vi "MIMIC Commands Rev 4.vi"(6 "MIMIC HOST COMMAND":T2(ring)=enum."Read Serial Number", 8 "Input String Data Array":string[](array[string])=["1"], 9 "HWHSflag":bool, 10 "wait (ms)":u32=500, 11 "VISA resource name":refnum<visa-resource-name>="COM5") -> (0 "error out":errorcluster={"status"=FALSE, "code"=1073676294, "source"="VISA Read in MIMIC RecvCommand.vi->MIMIC Commands Rev 2.vi"}, 1 "Receive_buffer":u8[](array[numeric]) format="%x", 2 "Receive_Unpacked_Data":T1)   [LabVIEW 2014]
panel:
  out "local":i32
  out "GUID":string
  out "Array":u8[](array[numeric]) format="%x"
  out "TimeToDecode":u16
  out "VISA resource name OUT":refnum<visa-resource-name>="COM5"
  out "hex integer string":string[](array[string])=["4", "D0", "0", "0", "FF", "2C"]
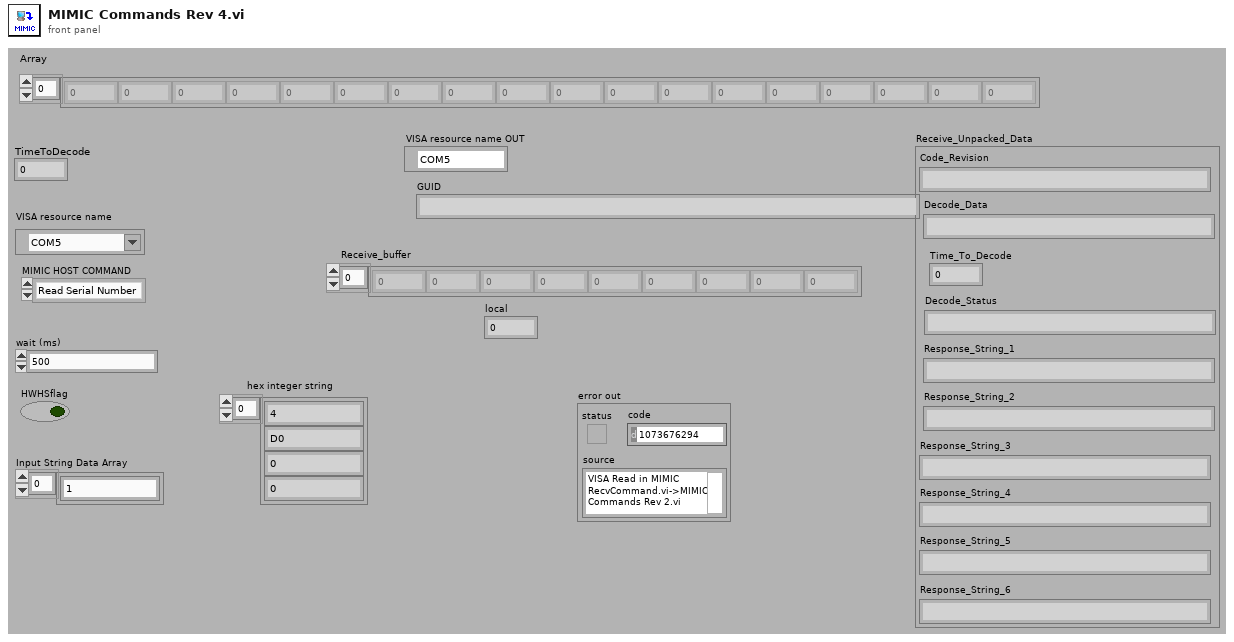
[diagram p1: front panel]
types:
  T1 = cluster{"Code_Revision":string, "Decode_Data":string, "Decode_Status":string, "Response_String_1":string, "Response_String_2":string, "Response_String_3":string, "Response_String_4":string, "Response_String_5":string, "Response_String_6":string, "Time_To_Decode":u16}
  T2 = enum16{"Enter FAT", "Beeper Control", "LED Off", "LED On", "Image Mode", "Start Session", "Stop Session", "Change Buadrate", "Auto Exposure", "Set Manual Exposure", "Read BT Address", "Store BT Address", "Pairing Command", "Query Paired Address", "Pairing Status", "Un-Pairing", "Set Illumination", "Trigger", "Set Defaults", "Imager Time To Decode Test", "Battery Off", "Battery Charge Control", "Read Battery Voltage", "Read Battery Temperature", "Software Version", "StoreFeatureSet", "ReadFeatureSet", "Store Model Number", "Read Model Number", "Store Manufacturing Date", "Read Manufacturing Date", "Store Service Date", "Read Service Date", "Store Serial Number", "Read Serial Number", "Exit FAT", "Read GUID", "Cable Auto ID", "Store RSM 627", "Read RSM 627", "Hall Effect switch", "Store GUID ", "ParamSend", "General", "General-Response", "RSM Init", "RSM EnterFAT", "RSM - SE4500 - Peek PRISM Register GENERIC command", "RSM - SE4500 - Poke PRISM Register GENERIC command", "RSM - SE4500 - GENERIC command", "RSM - SE4500 - GetPDM Calibration", "RSM - SE4500 - SetPDM Calibration", "Get Object Sensor Value", "Store Object Sensor Calibration Value", "Read Object Sensor Calibration Value", "RSM - SE4500 - GetPDM-Z Calibration", "RSM - SE4500 - SetPDM-Z Calibration"}
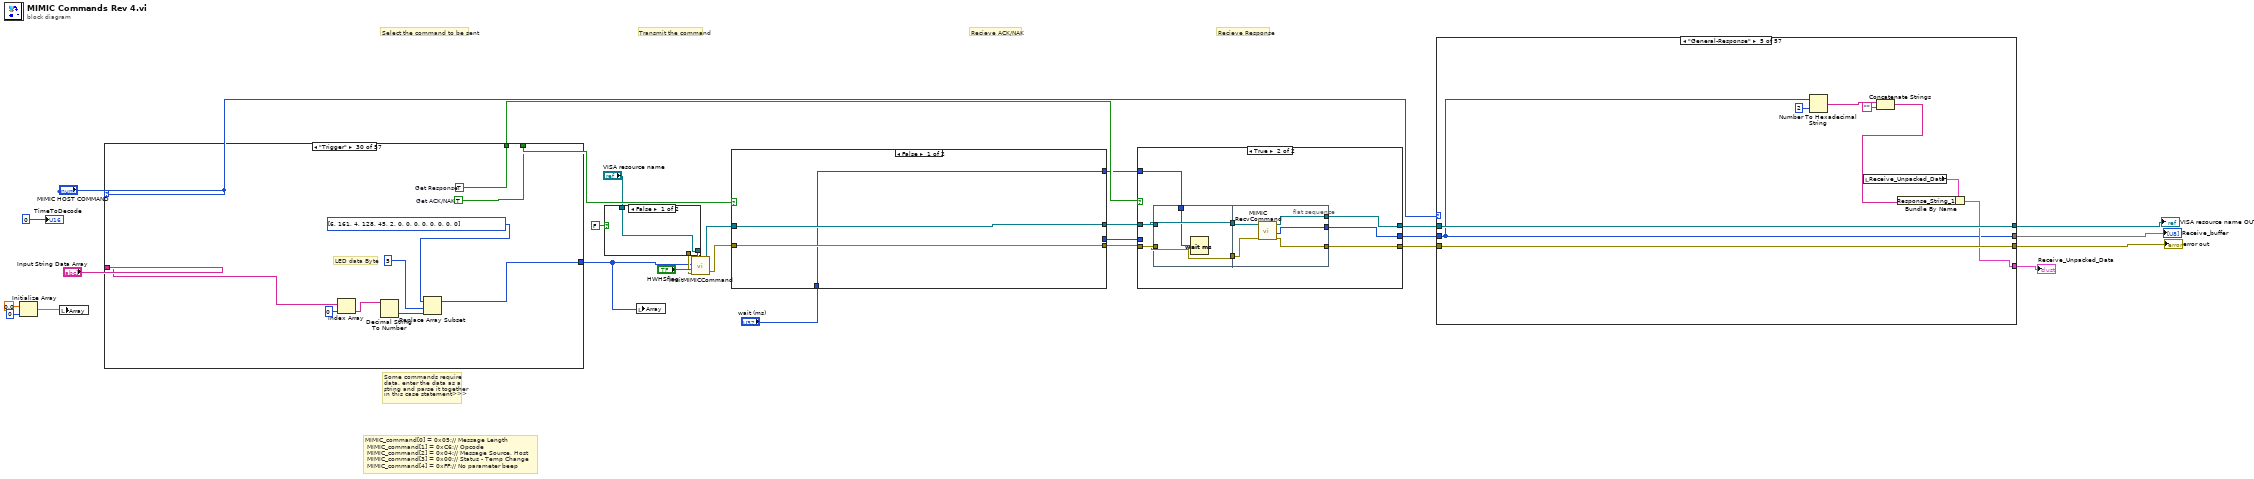
[diagram p0: block diagram]
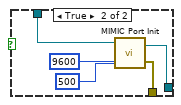
[diagram p2: hidden frame]
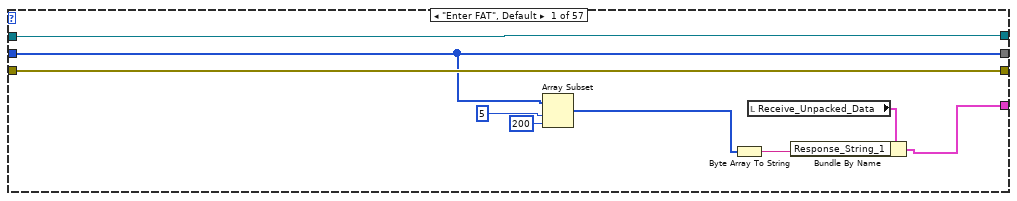
[diagram p3: hidden frame]
diagram:
  # "MIMIC_command[0] = 0x05;// Message Length \n\tMIMIC_command[1] = 0xC6;// Opcode  \n\tMIMIC_command[2] = 0x04;// Message Source, Host \n\tMIMIC_command[3] = 0x00;// Status - Temp Change            \n\tMIMIC_command[4] = 0xFF;// No parameter beep"
  # "Transmit the command"
  # "Recieve Response"
  # "Recieve ACK/NAK"
  # "Select the command to be sent"
  # "Some commands require\ndata, enter the data as a\nstring and parse it together\nin this case statement>>>"
  n1 = Initialize Array(0.0 ("element"), 0 ("dimension size")) -> (w5:dbl[])
  n2 = local write "Array"(w5) -> ()
  n3 = case shown="\"Trigger\"" "MIMIC HOST COMMAND" {
    tunnel: "Input String Data Array" -> [w37 w39 w62 _ _ _ _ _ w86 w113 w139 w179 w219 w256 _ _ _ w274 w290 w300 w313 w331 w347 _ _ _ _ _ w371 w379 _ _ w397 _ _ _ _ w422 _ w434 _ w444 _ _ _ w470 _ w482 _ _ _ _ _ _ _ _ _]
    tunnel: [w31 w45 w66 u8[] [5, 161, 4, 128, 16, 0, 0, 0, 0, 0, 0, 0, 0, 0] u8[] [14, 128, 4, 0, 0, 10, 112, 0, 1, 20, 112, 12, 0, 132] u8[] [14, 128, 4, 0, 0, 10, 112, 0, 1, 20, 112, 31, 0, 113] u8[] [12, 128, 4, 0, 0, 6, 32, 0, 0, 240, 0, 0, 0, 0] u8[] [13, 128, 4, 0, 0, 9, 112, 0, 1, 2, 120, 1, 135, 0] w85 w119 w140 w176 w217 w257 u8[] [4, 228, 4, 0, 0, 0, 0, 0, 0, 0, 0, 0, 0, 0] u8[] [4, 228, 4, 0, 0, 0, 0, 0, 0, 0, 0, 0, 0, 0] u8[] [7, 215, 4, 0, 4, 11, 0, 255, 15, 0, 0, 0, 0, 0] w275 w284 w298 w317 w334 w346 u8[] [16, 161, 4, 128, 16, 0, 0, 0, 0, 0, 0, 0, 0, 0] u8[] [5, 161, 4, 128, 16, 0, 0, 0, 0, 0, 0, 0, 0, 0] u8[] [4, 200, 4, 128, 0, 0, 0, 0, 0, 0, 0, 0, 0, 0] u8[] [5, 161, 4, 128, 25, 0, 0, 0, 0, 0, 0, 0, 0, 0] u8[] [7, 161, 4, 128, 66, 2, 29, 0, 0, 0, 0, 0, 0, 0] w370 w381 u8[] [7, 161, 4, 128, 48, 19, 136, 0, 0, 0, 0, 0, 0, 0] u8[] [5, 161, 4, 128, 60, 0, 0, 0, 0, 0, 0, 0, 0, 0] w396 u8[] [7, 161, 4, 128, 66, 117, 48, 0, 0, 0, 0, 0, 0, 0] u8[] [7, 161, 4, 128, 66, 117, 49, 0, 0, 0, 0, 0, 0, 0] u8[] [7, 161, 4, 128, 66, 78, 41, 0, 0, 0, 0, 0, 0, 0] u8[] [6, 161, 4, 128, 96, 8] w415 u8[] [7, 161, 4, 128, 66, 3, 36] w436 u8[] [7, 161, 4, 128, 66, 2, 194, 0, 0, 0, 0, 0, 0, 0] w449 u8[] [7, 161, 4, 128, 66, 2, 21, 0, 0, 0, 0, 0, 0, 0] w463 u8[] [7, 161, 4, 128, 66, 2, 23, 0, 0, 0, 0, 0, 0, 0] w475 u8[] [7, 161, 4, 128, 66, 2, 24, 0, 0, 0, 0, 0, 0, 0] w487 u8[] [7, 161, 4, 128, 66, 2, 22, 0, 0, 0, 0, 0, 0, 0] u8[] [5, 161, 4, 128, 54, 254, 160, 0, 0, 0, 0, 0, 0, 0] u8[] [5, 161, 4, 128, 84, 0, 0, 0, 0, 0, 0, 0, 0, 0] u8[] [5, 161, 4, 128, 47] w502 u8[] [5, 161, 4, 128, 110] u8[] [10, 161, 4, 128, 69, 2, 115, 66, 7, 2] u8[] [6, 161, 4, 128, 45, 1, 0, 0, 0, 0, 0, 0, 0, 0] u8[] [7, 161, 4, 128, 66, 2, 115]] -> w6
    tunnel: [w30 w57 w64 w71 w75 w78 w81 w84 w108 w135 w172 w192 w232 w258 w266 w269 w271 w276 w291 w301 w318 w335 w353 w356 w358 w361 w365 w369 w373 w386 w390 w393 w394 w405 w408 w410 w413 w428 w431 w439 w442 w448 w453 w462 w467 w474 w478 w485 w490 w494 w498 w499 w507 w509 w512 w515 w519] -> w25
    tunnel: [w29 w56 w65 w70 w74 w77 w80 w83 w107 w134 w171 w191 w231 w259 w267 w270 w272 w277 w292 w302 w319 w336 w354 w357 w359 w362 w364 w368 w372 w387 w389 w392 w395 w404 w407 w409 w412 w427 w430 w438 w441 w447 w454 w461 w466 w473 w479 w486 w491 w493 w497 w500 w508 w510 w513 w516 w518] -> w27
    frame "LED On" {
      w30 = FALSE  # Get Response
      w29 = TRUE  # Get ACK/NAK
      # "LED data Byte"
      n4 = Index Array(array=w37, index=0) -> (element=w36:string)
      n5 = Decimal String To Number(string=w36) -> (number=w35:i32)  [unwired: 2 in, 1 out]
      n6 = Replace Array Subset(array=u8[] [5, 231, 4, 128, 1, 0, 0, 0, 0, 0, 0, 0, 0, 0], new element=w35, index=4) -> (w31:u8[])
    }
    frame "ParamSend" {
      w57 = FALSE  # Get Response
      w56 = TRUE  # Get ACK/NAK
      n7 = Array Size(array=w39) -> (size(s)=w38:i32)
      n8 = Index Array(array=w39, index=0) -> (element=w61:string)
      n9 = Add(x=w38, y=5) -> (x+y=w43:i32)
      n10 = Hexadecimal String To Number(string=w61) -> (number=w42:u32)  [unwired: 2 in, 1 out]
      n11 = Replace Array Subset(array=u8[] [5, 198, 4, 128, 255, 0, 0, 0, 0, 0, 0, 0, 0, 0], new element=w43, index=0) -> (w54:u8[])
      n12 = Replace Array Subset(array=w54, new element=w42, index=5) -> (w50:u8[])
      n13 = Index Array(array=w39, index=2) -> (element=w49:string)
      n14 = Index Array(array=w39, index=1) -> (element=w53:string)
      n15 = Hexadecimal String To Number(string=w49) -> (number=w40:u32)  [unwired: 2 in, 1 out]
      n16 = Hexadecimal String To Number(string=w53) -> (number=w41:u32)  [unwired: 2 in, 1 out]
      n17 = Replace Array Subset(array=w50, new element=w41, index=6) -> (w46:u8[])
      n18 = Replace Array Subset(array=w46, new element=w40, index=7) -> (w45:u8[])
    }
    frame "Beeper Control" {
      w64 = FALSE  # Get Response
      w65 = TRUE  # Get ACK/NAK
      # "Beeper data Byte"
      n19 = Decimal String To Number(string=w62, offset=0) -> (number=w69:i32[])  [unwired: 1 in, 1 out]
      n20 = Replace Array Subset(array=u8[] [5, 230, 4, 128, 0, 0, 0, 0, 0, 0, 0, 0, 0, 0], new element=w69, index=4) -> (w66:u8[])
    }
    frame "Enter FAT" {
      w71 = TRUE  # Get Response
      w70 = TRUE  # Get ACK/NAK
      # "Enter FAT command:\n0x05:0xA1:0x40:0x80:0x10"
    }
    frame "RSM - SE4500 - GetPDM Calibration" {
      w75 = TRUE  # Get Response
      w74 = FALSE  # Get ACK/NAK
      # "RSM GetDPMCalibration Command"
    }
    frame "RSM - SE4500 - GetPDM-Z Calibration" {
      w78 = TRUE  # Get Response
      w77 = FALSE  # Get ACK/NAK
      # "RSM GetDPMCalibration Command"
    }
    frame "RSM Init" {
      w81 = TRUE  # Get Response
      w80 = FALSE  # Get ACK/NAK
      # "Init RSM command:\n0x0C:0x80:0x04:0x00:0x00:0x06:0x20:0x00:0x00:0xF0"
    }
    frame "RSM EnterFAT" {
      w84 = TRUE  # Get Response
      w83 = FALSE  # Get ACK/NAK
      # "RSM / SE4500 - Enter FAT command:\n0x0D:0x80:0x04:0x00:0x00:0x09:0x70:0x00:0x01:0x02:0x78:0x01:0x87:"
    }
    frame "RSM - SE4500 - Peek PRISM Register GENERIC command" {
      w108 = TRUE  # Get Response
      w107 = FALSE  # Get ACK/NAK
      # "Register Word - HEX String"
      # "RSM / SE4500 - Peek PRISM Register GENERIC command:\n0x0E:0x80:0x04:0x00:0x00:0x0B:0x70:0x00:0x01:0x02:0xC3:0xXX:0xXX:0xXX:0xCS"
      n21 = Index Array(array=w86, index=0) -> (element=w90:string)
      n22 = Hexadecimal String To Number(string=w90, default (0uL)=i16 0 ("default (0 I32)")) -> (number=w88:i16)  [unwired: 1 in, 1 out]
      n23 = Split Number(x=w88) -> (hi(x)=w94:u8, lo(x)=w92:u8)
      n24 = Replace Array Subset(array=u8[] [15, 128, 4, 0, 0, 11, 112, 0, 1, 3, 195, 0, 0, 0, 0], new element=w94, index=11) -> (w91:u8[])
      n25 = Replace Array Subset(array=w91, new element=w92, index=12) -> (w87:u8[])
      n26 = Array Subset(array=w87, index=10, length=3) -> (w97:u8[])
      n27 = for {
        N: 3 -> [_]
        tunnel: w97 -> [w111] mode=indexing
        shift-right: [w109] -> w103
        shift-left: u16 0 -> [w110]
        n28 = Add(x=w110, y=w111) -> (x+y=w109:u16)
      }
      n29 = Not(x=w103) -> (.not. x?=w102:u16)
      n30 = Increment(x=w102) -> (x+1=w101:u16)
      n31 = Replace Array Subset(array=w87, new element=w101, index=13) -> (w85:u8[])
    }
    frame "RSM - SE4500 - GENERIC command" {
      w114 = 1 ("index")
      w118 = 0 ("index")
      w135 = TRUE  # Get Response
      w134 = FALSE  # Get ACK/NAK
      # "Register Word - HEX String"
      # "RSM / SE4500 - Peek PRISM Register GENERIC command:\n0x0E:0x80:0x04:0x00:0x00:0x0B:0x70:0x00:0x01:0x02:0xXX:0xXX:0xXX:0xCS"
      n32 = Index Array(array=w113, index=w118) -> (element=w121:string)
      n33 = Index Array(array=w113, index=w114) -> (element=w115:string)
      n34 = Hexadecimal String To Number(string=w121, default (0uL)=w118) -> (number=w116:i32)  [unwired: 1 in, 1 out]
      n35 = Hexadecimal String To Number(string=w115, default (0uL)=w114) -> (number=w112:i32)  [unwired: 1 in, 1 out]
      n36 = Replace Array Subset(array=u8[] [13, 128, 4, 0, 0, 9, 112, 0, 1, 2, 255, 0, 0], new element=w116, index=10) -> (w122:u8[])
      n37 = Replace Array Subset(array=w122, new element=w112, index=11) -> (w120:u8[])
      n38 = Array Subset(array=w120, index=10, length=2) -> (w125:u8[])
      n39 = for {
        N: 2 -> [_]
        tunnel: w125 -> [w138] mode=indexing
        shift-right: [w136] -> w131
        shift-left: u16 0 -> [w137]
        n40 = Add(x=w137, y=w138) -> (x+y=w136:u16)
      }
      n41 = Not(x=w131) -> (.not. x?=w130:u16)
      n42 = Increment(x=w130) -> (x+1=w129:u16)
      n43 = Replace Array Subset(array=w120, new element=w129, index=12) -> (w119:u8[])
    }
    frame "RSM - SE4500 - Poke PRISM Register GENERIC command" {
      w172 = TRUE  # Get Response
      w171 = FALSE  # Get ACK/NAK
      # "Register Word - HEX String"
      # "Register Word - HEX String"
      # "Value Byte - Decimal String"
      # "RSM / SE4500 - Poke PRISM Register GENERIC command:\n0x0E:0x80:0x04:0x00:0x00:0x0B:0x70:0x00:0x01:0x02:0xC0:0xXX:0xXX:0xXX:0xCS"
      n44 = Index Array(array=w139, index=0) -> (element=w154:string)
      n45 = Index Array(array=w139, index=1) -> (element=w145:string)
      n46 = Hexadecimal String To Number(string=w154, default (0uL)=i16 0 ("default (0 I32)")) -> (number=w152:i16)  [unwired: 1 in, 1 out]
      n47 = Split Number(x=w152) -> (hi(x)=w158:u8, lo(x)=w156:u8)
      n48 = Hexadecimal String To Number(string=w145, default (0uL)=i16 0 ("default (0 I32)")) -> (number=w151:i16)  [unwired: 1 in, 1 out]
      n49 = Replace Array Subset(array=u8[] [16, 128, 4, 0, 0, 12, 112, 0, 1, 2, 151, 0, 0, 0, 0, 0], new element=w158, index=12) -> (w155:u8[])
      n50 = Split Number(x=w151) -> (hi(x)=w148:u8, lo(x)=w150:u8)
      n51 = Replace Array Subset(array=w155, new element=w156, index=11) -> (w143:u8[])
      n52 = Replace Array Subset(array=w143, new element=w148, index=14) -> (w142:u8[])
      n53 = Replace Array Subset(array=w142, new element=w150, index=13) -> (w141:u8[])
      n54 = Array Subset(array=w141, index=10, length=5) -> (w161:u8[])
      n55 = for {
        N: 5 -> [_]
        tunnel: w161 -> [w175] mode=indexing
        shift-right: [w173] -> w167
        shift-left: u16 0 -> [w174]
        n56 = Add(x=w174, y=w175) -> (x+y=w173:u16)
      }
      n57 = Not(x=w167) -> (.not. x?=w166:u16)
      n58 = Increment(x=w166) -> (x+1=w165:u16)
      n59 = Replace Array Subset(array=w141, new element=w165, index=15) -> (w140:u8[])
    }
    frame "RSM - SE4500 - SetPDM Calibration" {
      w192 = TRUE  # Get Response
      w191 = FALSE  # Get ACK/NAK
      # "RSM / SE4500 - SetDPMCalibration command:"
      n60 = for {
        N: 8 -> [_]
        shift-right: [w202] -> w178
        shift-left: u8[] [30, 128, 4, 0, 0, 26, 112, 0, 1, 2, 148, 12, 0, 0, 0, 0, 0, 0, 0, 0, 0, 0, 0, 0, 0, 0, 0, 0, 0, 0, 0] -> [w209]
        tunnel: w179 -> [w208]
        i -> [w204]
        # "high byte"
        # "low byte"
        n61 = Index Array(array=w208, index=w204) -> (element=w197:string)
        n62 = Decimal String To Number(string=w197, default (0L)=0 ("default (0 I32)")) -> (number=w194:i32)  [unwired: 1 in, 1 out]
        n63 = Number To Hexadecimal String(1:i16 4 ("width (-)"), 2:w194) -> (0:w195:string)
        n64 = local read "local"() -> (w200:i32)
        n65 = Hexadecimal String To Number(string=w195, default (0uL)=i16 0 ("default (0 I32)")) -> (number=w210:i16)  [unwired: 1 in, 1 out]
        n66 = Add(x=1 ("y"), y=w200) -> (x+y=w198:i32)
        n67 = Add(x=w204, y=w198) -> (x+y=w201:i32)
        n68 = Add(x=1 ("index"), y=w201) -> (x+y=w206:i32)
        n69 = Split Number(x=w210) -> (hi(x)=w212:u8, lo(x)=w211:u8)
        n70 = Replace Array Subset(array=w209, new element=w212, index=w206) -> (w203:u8[])
        n71 = local write "local"(w198) -> ()
        n72 = Replace Array Subset(array=w203, new element=w211, index=w201) -> (w202:u8[])
      }
      n73 = Array Subset(array=w178, index=10, length=19) -> (w182:u8[])
      n74 = for {
        N: 19 -> [_]
        tunnel: w182 -> [w215] mode=indexing
        shift-right: [w213] -> w188
        shift-left: u16 0 -> [w214]
        n75 = Add(x=w214, y=w215) -> (x+y=w213:u16)
      }
      n76 = Not(x=w188) -> (.not. x?=w187:u16)
      n77 = Increment(x=w187) -> (x+1=w186:u16)
      n78 = Replace Array Subset(array=w178, new element=w186, index=29) -> (w176:u8[])
      "local" <- 12 ("x+y")
    }
    frame "RSM - SE4500 - SetPDM-Z Calibration" {
      w232 = TRUE  # Get Response
      w231 = FALSE  # Get ACK/NAK
      # "RSM / SE4500 - SetDPMCalibration command:"
      n79 = local write "local"(12 ("x+y")) -> ()
      n80 = for {
        N: 8 -> [_]
        shift-right: [w242] -> w218
        shift-left: u8[] [30, 128, 4, 0, 0, 26, 112, 0, 1, 2, 148, 31, 0, 0, 0, 0, 0, 0, 0, 0, 0, 0, 0, 0, 0, 0, 0, 0, 0, 0, 0] -> [w249]
        tunnel: w219 -> [w248]
        i -> [w244]
        # "high byte"
        # "low byte"
        n81 = Index Array(array=w248, index=w244) -> (element=w237:string)
        n82 = Decimal String To Number(string=w237, default (0L)=0 ("default (0 I32)")) -> (number=w234:i32)  [unwired: 1 in, 1 out]
        n83 = Number To Hexadecimal String(1:i16 4 ("width (-)"), 2:w234) -> (0:w235:string)
        n84 = local read "local"() -> (w240:i32)
        n85 = Hexadecimal String To Number(string=w235, default (0uL)=i16 0 ("default (0 I32)")) -> (number=w250:i16)  [unwired: 1 in, 1 out]
        n86 = Add(x=1 ("y"), y=w240) -> (x+y=w238:i32)
        n87 = Add(x=w244, y=w238) -> (x+y=w241:i32)
        n88 = Add(x=1 ("index"), y=w241) -> (x+y=w246:i32)
        n89 = Split Number(x=w250) -> (hi(x)=w252:u8, lo(x)=w251:u8)
        n90 = Replace Array Subset(array=w249, new element=w252, index=w246) -> (w243:u8[])
        n91 = local write "local"(w238) -> ()
        n92 = Replace Array Subset(array=w243, new element=w251, index=w241) -> (w242:u8[])
      }
      n93 = Array Subset(array=w218, index=10, length=19) -> (w222:u8[])
      n94 = for {
        N: 19 -> [_]
        tunnel: w222 -> [w255] mode=indexing
        shift-right: [w253] -> w228
        shift-left: u16 0 -> [w254]
        n95 = Add(x=w254, y=w255) -> (x+y=w253:u16)
      }
      n96 = Not(x=w228) -> (.not. x?=w227:u16)
      n97 = Increment(x=w227) -> (x+1=w226:u16)
      n98 = Replace Array Subset(array=w218, new element=w226, index=29) -> (w217:u8[])
    }
    frame "Image Mode" {
      w258 = FALSE  # Get Response
      w259 = TRUE  # Get ACK/NAK
      # "Image Mode Byte:\n00: Decode\n01: SnapShot\n02: Video\n03: Last Decode\n04: las No Decode"
      n99 = Index Array(array=w256, index=0) -> (element=w264:string)
      n100 = Decimal String To Number(string=w264) -> (number=w263:i32)  [unwired: 2 in, 1 out]
      n101 = Replace Array Subset(array=u8[] [5, 247, 4, 128, 0, 0, 0, 0, 0, 0, 0, 0, 0, 0], new element=w263, index=4) -> (w257:u8[])
    }
    frame "Start Session" {
      w266 = FALSE  # Get Response
      w267 = TRUE  # Get ACK/NAK
      # "Start Session"
    }
    frame "Stop Session" {
      w269 = FALSE  # Get Response
      w270 = TRUE  # Get ACK/NAK
      # "Start Session"
    }
    frame "Change Buadrate" {
      w271 = FALSE  # Get Response
      w272 = FALSE  # Get ACK/NAK
      # "Enter FAT command:\n06: 9600\n08: 38400\n0A: 57600\n0B:115200\n0C:230400"
    }
    frame "Auto Exposure" {
      w276 = FALSE  # Get Response
      w277 = TRUE  # Get ACK/NAK
      # "Auto Exposure:\n00:Disabled\n01: Enabled"
      n102 = Index Array(array=w274, index=0) -> (element=w282:string)
      n103 = Decimal String To Number(string=w282) -> (number=w281:i32)  [unwired: 2 in, 1 out]
      n104 = Replace Array Subset(array=u8[] [8, 198, 4, 0, 255, 240, 41, 0, 0, 0, 0, 0, 0, 0], new element=w281, index=7) -> (w275:u8[])
    }
    frame "Set Manual Exposure" {
      w291 = FALSE  # Get Response
      w292 = TRUE  # Get ACK/NAK
      # "Image Mode Byte:\n00: Decode\n01: SnapShot\n02: Video\n03: Last Decode\n04: las No Decode"
      n105 = Index Array(array=w290, index=0) -> (element=w296:string)
      n106 = Decimal String To Number(string=w296, default (0L)=u16 0 ("default (0 I32)")) -> (number=w289:u16)  [unwired: 1 in, 1 out]
      n107 = Split Number(x=w289) -> (hi(x)=w287:u8, lo(x)=w286:u8)
      n108 = Replace Array Subset(array=u8[] [10, 198, 4, 0, 255, 244, 241, 55, 0, 0, 0, 0, 0, 0], new element=w287, index=8) -> (w283:u8[])
      n109 = Replace Array Subset(array=w283, new element=w286, index=9) -> (w284:u8[])
    }
    frame "Store BT Address" {
      w301 = FALSE  # Get Response
      w302 = TRUE  # Get ACK/NAK
      # "Store BT command:\n0x16, 0xA1, 0x04, 0x80, 0x45, 0x02, 0x1D, 0x41, 0x07, 0x42, 0x00, 0x06, 0x00, 0x00, \n\t\t\t\t\t\t\t\t\t\t0x00, 0x00, 0x00, 0x00, 0x00, 0x00,0x00, 0x00, 0xFF, 0xFF};"
      n110 = for {
        N: 6 -> [_]
        tunnel: w300 -> [w311]
        tunnel: [w306] -> w298
        i -> [w308]
        n111 = Index Array(array=w311, index=w308) -> (element=w305:string)
        n112 = Add(x=14 ("index"), y=w308) -> (x+y=w309:i32)
        n113 = Hexadecimal String To Number(string=w305, offset=0) -> (number=w303:u32)  [unwired: 1 in, 1 out]
        n114 = local read "Array"() -> (w307:u8[])
        n115 = Replace Array Subset(array=w307, new element=w303, index=w309) -> (w306:u8[])
        n116 = local write "Array"(w306) -> ()
      }
      "Array" <- u8[] [22, 161, 4, 128, 69, 2, 29, 65, 7, 66, 0, 6, 0, 0, 0, 0, 0, 0, 0, 0, 255, 255, 255, 0, 0, 0]
    }
    frame "General" {
      w315 = 0 ("offset")
      w318 = FALSE  # Get Response
      w319 = TRUE  # Get ACK/NAK
      # "Gneral FAT command:\n0x16, 0xA1, 0x04, 0x80, 0x45, 0x02, 0x1D, 0x41, 0x07, 0x42, 0x00, 0x06, 0x00, 0x00, \n\t\t\t\t\t\t\t\t\t\t0x00, 0x00, 0x00, 0x00, 0x00, 0x00,0x00, 0x00, 0xFF, 0xFF};"
      n117 = Index Array(array=w313, index=w315) -> (element=w314:string)
      n118 = Hexadecimal String To Number(string=w314, offset=w315) -> (number=w312:u32)  [unwired: 1 in, 1 out]
      n119 = for {
        N: w312 -> [_]
        tunnel: w313 -> [w328]
        tunnel: [w323] -> w317
        i -> [w325]
        n120 = Index Array(array=w328, index=w325) -> (element=w322:string)
        n121 = Add(x=0 ("index"), y=w325) -> (x+y=w326:i32)
        n122 = Hexadecimal String To Number(string=w322, offset=0) -> (number=w320:u32)  [unwired: 1 in, 1 out]
        n123 = local read "Array"() -> (w324:u8[])
        n124 = Replace Array Subset(array=w324, new element=w320, index=w326) -> (w323:u8[])
        n125 = local write "Array"(w323) -> ()
      }
      n126 = local write "Array"(u8[] [22, 0, 0, 0, 0, 0, 0, 0, 0, 0, 0, 0, 0, 0, 0, 0, 0, 0, 0, 0, 0, 0, 0, 0, 0, 0]) -> ()
    }
    frame "General-Response" {
      w330 = 0 ("offset")
      w335 = TRUE  # Get Response
      w336 = TRUE  # Get ACK/NAK
      # "Gneral FAT command:\n0x16, 0xA1, 0x04, 0x80, 0x45, 0x02, 0x1D, 0x41, 0x07, 0x42, 0x00, 0x06, 0x00, 0x00, \n\t\t\t\t\t\t\t\t\t\t0x00, 0x00, 0x00, 0x00, 0x00, 0x00,0x00, 0x00, 0xFF, 0xFF};"
      n127 = Index Array(array=w331, index=w330) -> (element=w329:string)
      n128 = Hexadecimal String To Number(string=w329, offset=w330) -> (number=w332:u32)  [unwired: 1 in, 1 out]
      n129 = for {
        N: w332 -> [_]
        tunnel: w331 -> [w345]
        tunnel: [w340] -> w334
        i -> [w342]
        n130 = Index Array(array=w345, index=w342) -> (element=w339:string)
        n131 = Add(x=0 ("index"), y=w342) -> (x+y=w343:i32)
        n132 = Hexadecimal String To Number(string=w339, offset=0) -> (number=w337:u32)  [unwired: 1 in, 1 out]
        n133 = local read "Array"() -> (w341:u8[])
        n134 = Replace Array Subset(array=w341, new element=w337, index=w343) -> (w340:u8[])
        n135 = local write "Array"(w340) -> ()
      }
      n136 = local write "Array"(u8[] [22, 0, 0, 0, 0, 0, 0, 0, 0, 0, 0, 0, 0, 0, 0, 0, 0, 0, 0, 0, 0, 0, 0, 0, 0, 0]) -> ()
    }
    frame "Pairing Command" {
      w353 = TRUE  # Get Response
      w354 = FALSE  # Get ACK/NAK
      # "Pairing  command:\n10 9E 04 80 00 00 02 03 06 08  01 0B 03 00 0F 0F FE 8E"
      n137 = Index Array(array=w347, index=0) -> (element=w351:string)
      n138 = String To Byte Array(string=w351) -> (unsigned byte array=w349:u8[])
      n139 = Replace Array Subset(array=u8[] [16, 158, 4, 128, 0, 0, 0, 0, 0, 8, 1, 11, 3, 0, 15, 15], new element=w349, index=4) -> (w346:u8[])
    }
    frame "Un-Pairing" {
      w356 = TRUE  # Get Response
      w357 = FALSE  # Get ACK/NAK
      # "Enter FAT command:\n0x05:0xA1:0x40:0x80:0x10"
    }
    frame "Set Illumination" {
      w358 = TRUE  # Get Response
      w359 = FALSE  # Get ACK/NAK
      # "Enter FAT command:\n0x05:0xA1:0x40:0x80:0x10"
    }
    frame "Set Defaults" {
      w361 = FALSE  # Get Response
      w362 = TRUE  # Get ACK/NAK
    }
    frame "Exit FAT" {
      w365 = TRUE  # Get Response
      w364 = TRUE  # Get ACK/NAK
    }
    frame "Read BT Address" {
      w369 = TRUE  # Get Response
      w368 = TRUE  # Get ACK/NAK
    }
    frame "LED Off" {
      w373 = FALSE  # Get Response
      w372 = TRUE  # Get ACK/NAK
      # "LED data Byte"
      n140 = Index Array(array=w371, index=0) -> (element=w378:string)
      n141 = Decimal String To Number(string=w378) -> (number=w377:i32)  [unwired: 2 in, 1 out]
      n142 = Replace Array Subset(array=u8[] [5, 232, 4, 128, 1, 0, 0, 0, 0, 0, 0, 0, 0, 0], new element=w377, index=4) -> (w370:u8[])
    }
    frame "Trigger" {
      w386 = TRUE  # Get Response
      w387 = TRUE  # Get ACK/NAK
      # "LED data Byte"
      n143 = Index Array(array=w379, index=0) -> (element=w385:string)
      n144 = Decimal String To Number(string=w385) -> (number=w384:i32)  [unwired: 2 in, 1 out]
      n145 = Replace Array Subset(array=u8[] [6, 161, 4, 128, 45, 2, 0, 0, 0, 0, 0, 0, 0, 0], new element=w384, index=5) -> (w381:u8[])
    }
    frame "Imager Time To Decode Test" {
      w390 = TRUE  # Get Response
      w389 = TRUE  # Get ACK/NAK
      # "Start Session"
    }
    frame "Battery Off" {
      w393 = FALSE  # Get Response
      w392 = TRUE  # Get ACK/NAK
      # "Enter FAT command:\n0x05:0xA1:0x40:0x80:0x10"
    }
    frame "Battery Charge Control" {
      w394 = FALSE  # Get Response
      w395 = TRUE  # Get ACK/NAK
      # "Battery Charge\n0x06, 0xA1, 0x04, 0x80, 0x3D\n0x00: Disable charging of battery\n0x01: Enable charging of battery\n0x02: Enable Slow charge (Hammer)"
      n146 = Index Array(array=w397, index=0) -> (element=w402:string)
      n147 = Decimal String To Number(string=w402) -> (number=w401:i32)  [unwired: 2 in, 1 out]
      n148 = Replace Array Subset(array=u8[] [6, 161, 4, 128, 61, 0, 0, 0, 0, 0, 0, 0, 0, 0], new element=w401, index=5) -> (w396:u8[])
    }
    frame "Read Battery Voltage" {
      w405 = TRUE  # Get Response
      w404 = FALSE  # Get ACK/NAK
      # "Read Battery Voltage command:\n0x07:0xA1:0x04:0x80:0x42:0x75:0x30"
    }
    frame "Read Battery Temperature" {
      w408 = TRUE  # Get Response
      w407 = FALSE  # Get ACK/NAK
      # "Read Battery Temperature command:\n0x07:0xA1:0x04:0x80:0x42:0x75:0x31"
    }
    frame "Software Version" {
      w410 = TRUE  # Get Response
      w409 = TRUE  # Get ACK/NAK
      # "Software Version command:\n\"0x07, 0xA1, 0x04, 0x80, 0x42, 0x4E, 0x29,\""
    }
    frame "Get Object Sensor Value" {
      w413 = TRUE  # Get Response
      w412 = TRUE  # Get ACK/NAK
      # "Get Object Sensor command:\n\"0x06,0xA1,0x04,0x80,0x60,0x08,\""
    }
    frame "Store Object Sensor Calibration Value" {
      w428 = FALSE  # Get Response
      w427 = TRUE  # Get ACK/NAK
      # "Store Object Sensor Calibration command:\n\"0x0B,0xA1,0x04,0x80,0x45,0x03,0x24,0x57,0x07,CAL H,CAL L"
      n149 = Index Array(array=w422, index=1) -> (element=w417:string)
      n150 = Index Array(array=w422, index=0) -> (element=w425:string)
      n151 = Hexadecimal String To Number(string=w425) -> (number=w418:u32)  [unwired: 2 in, 1 out]
      n152 = Hexadecimal String To Number(string=w417) -> (number=w416:u32)  [unwired: 2 in, 1 out]
      n153 = Replace Array Subset(array=u8[] [11, 161, 4, 128, 69, 3, 36, 87, 7, 0, 0], new element=w418, index=9) -> (w420:u8[])
      n154 = Replace Array Subset(array=w420, new element=w416, index=10) -> (w415:u8[])
    }
    frame "Read Object Sensor Calibration Value" {
      w431 = TRUE  # Get Response
      w430 = TRUE  # Get ACK/NAK
      # "Read Object Sensor Calibration command:\n\"0x07,0xA1,0x04,0x80,0x42,0x03,0x24,\""
    }
    frame "StoreFeatureSet" {
      w439 = FALSE  # Get Response
      w438 = TRUE  # Get ACK/NAK
      # "Store Feature Set command:\n\"0x0A, 0xA1, 0x04, 0x80, 0x45, 0x02, 0xC2, 0x42, 0x07,\n0xFF,//Feature Set Value \n0x00, 0x00}; //checksum\""
      n155 = Hexadecimal String To Number(string=w434, offset=0) -> (number=w432:u32[])  [unwired: 1 in, 1 out]
      n156 = Replace Array Subset(array=u8[] [10, 161, 4, 128, 69, 2, 194, 66, 7, 0, 0, 0, 0, 0], new element=w432, index=9) -> (w436:u8[])
    }
    frame "ReadFeatureSet" {
      w442 = TRUE  # Get Response
      w441 = TRUE  # Get ACK/NAK
      # "0x07, 0xA1, 0x04, 0x80, 0x42, 0x02, 0xC2, 0x00, 0x00};"
      # "Read Feature Set command:\n0x07, 0xA1, 0x04, 0x80, 0x42, 0x02, 0xC2,"
    }
    frame "Store Model Number" {
      w448 = FALSE  # Get Response
      w447 = TRUE  # Get ACK/NAK
      # "StoreModel Number command:\n0x20, 0xA1, 0x04, 0x80, 0x45, 0x02, 0x15, 0x53, 0x07, 0x00, 0x12, 0x00, 0x00,\n\t\t\t\t\t\t\t\t\t\t0x00, 0x00, 0x00, 0x00, 0x00, 0x00, 0x00, 0x00, 0x00,\n\t\t\t\t\t\t\t\t\t\t0x00, 0x00, 0x00, 0x00, 0x00, 0x00, 0x00, 0x00, 0x00,\n\t\t\t\t\t\t\t\t\t\t0x00"
      n157 = Index Array(array=w444, index=0) -> (element=w445:string)
      n158 = String To Byte Array(string=w445) -> (unsigned byte array=w446:u8[])
      n159 = Replace Array Subset(array=u8[] [32, 161, 4, 128, 69, 2, 21, 83, 7, 0, 18, 0, 0, 0, 0, 0, 0, 0, 0, 0, 0, 0, 0, 0, 0, 0, 0, 0, 0, 0, 0, 0, 0], new element=w446, index=13) -> (w449:u8[])
    }
    frame "Read Model Number" {
      w453 = TRUE  # Get Response
      w454 = TRUE  # Get ACK/NAK
      # "ReadModel Number command:\n0x07, 0xA1, 0x04, 0x80, 0x42, 0x02, 0x15,"
    }
    frame "Store Manufacturing Date" {
      w462 = FALSE  # Get Response
      w461 = TRUE  # Get ACK/NAK
      # "Store Manufacturing Date command:\n0x15, 0xA1, 0x04, 0x80, 0x45, 0x02, 0x17, 0x53, 0x07, 0x00, 0x07, 0x00, 0x00,\n\t\t\t\t\t\t\t\t\t\t0x00, 0x00, 0x00, 0x00, 0x00, 0x00, 0x00,\n\t\t\t\t\t\t\t\t\t\t0x00"
      n160 = Get Date/Time In Seconds() -> (seconds since 1Jan1904=w460:timestamp)
      n161 = Format Date/Time String(time format string (%c)="%d%b%y", seconds (now)=w460, UTC format=FALSE) -> (date/time string=w456:string)
      n162 = To Upper Case(1:w456) -> (0:w455:string)
      n163 = String To Byte Array(string=w455) -> (unsigned byte array=w457:u8[])
      n164 = Replace Array Subset(array=u8[] [21, 161, 4, 128, 69, 2, 23, 83, 7, 0, 7, 0, 0, 0, 0, 0, 0, 0, 0, 0, 0, 0], new element=w457, index=13) -> (w463:u8[])
    }
    frame "Read Manufacturing Date" {
      w467 = TRUE  # Get Response
      w466 = TRUE  # Get ACK/NAK
      # "Read Feature Set command:\n0x07, 0xA1, 0x04, 0x80, 0x42, 0x02, 0x17,"
    }
    frame "Store Service Date" {
      w474 = FALSE  # Get Response
      w473 = TRUE  # Get ACK/NAK
      # "StoreService Date command:\n0x15, 0xA1, 0x04, 0x80, 0x45, 0x02, 0x18, 0x53, 0x07, 0x00, 0x07, 0x00, 0x00,\n\t\t\t\t\t\t\t\t\t\t0x00, 0x00, 0x00, 0x00, 0x00, 0x00, 0x00,\n\t\t\t\t\t\t\t\t\t\t0x00"
      n165 = Index Array(array=w470, index=0) -> (element=w472:string)
      n166 = String To Byte Array(string=w472) -> (unsigned byte array=w469:u8[])
      n167 = Replace Array Subset(array=u8[] [21, 161, 4, 128, 69, 2, 24, 83, 7, 0, 7, 0, 0, 0, 0, 0, 0, 0, 0, 0, 0, 0], new element=w469, index=13) -> (w475:u8[])
    }
    frame "Read Service Date" {
      w478 = TRUE  # Get Response
      w479 = TRUE  # Get ACK/NAK
      # "Read Service Date command:\n0x07, 0xA1, 0x04, 0x80, 0x42, 0x02, 0x18,"
    }
    frame "Store Serial Number" {
      w485 = FALSE  # Get Response
      w486 = TRUE  # Get ACK/NAK
      # "Store Serial Number command:\n0x1E, 0xA1, 0x04, 0x80, 0x45, 0x02, 0x16, 0x53, 0x07, 0x00, 0x10, 0x00, 0x00,\n\t\t\t\t\t\t\t\t\t\t0x00, 0x00, 0x00, 0x00, 0x00, 0x00, 0x00, 0x00,\n\t\t\t\t\t\t\t\t\t\t0x00, 0x00, 0x00, 0x00, 0x00, 0x00, 0x00, 0x00,\n\t\t\t\t\t\t\t\t\t\t0x00"
      n168 = Index Array(array=w482, index=0) -> (element=w484:string)
      n169 = String To Byte Array(string=w484) -> (unsigned byte array=w481:u8[])
      n170 = Replace Array Subset(array=u8[] [30, 161, 4, 128, 69, 2, 22, 83, 7, 0, 16, 0, 0, 0, 0, 0, 0, 0, 0, 0, 0, 0, 0, 0, 0, 0, 0, 0, 0, 0, 0, 0, 0], new element=w481, index=13) -> (w487:u8[])
    }
    frame "Read Serial Number" {
      w490 = TRUE  # Get Response
      w491 = TRUE  # Get ACK/NAK
      # "Read Serial Number command:\n0x07, 0xA1, 0x04, 0x80, 0x42, 0x02, 0x16,"
    }
    frame "Pairing Status" {
      w494 = TRUE  # Get Response
      w493 = FALSE  # Get ACK/NAK
      # "Read Serial Number command:\n0x05, 0xA1, 0x04, 0x80, 0x36, 0xFE, 0xA0,"
    }
    frame "Query Paired Address" {
      w498 = TRUE  # Get Response
      w497 = FALSE  # Get ACK/NAK
      # "Read Serial Number command:\n0x05, 0xA1, 0x04, 0x80, 0x54,"
    }
    frame "Read GUID" {
      w499 = TRUE  # Get Response
      w500 = TRUE  # Get ACK/NAK
      # "\"0x05, 0xA1, 0x04, 0x80, 0x2F,\""
    }
    frame "Store GUID " {
      w507 = TRUE  # Get Response
      w508 = FALSE  # Get ACK/NAK
      # "32 bytes 0-9, A-F (0x30 - 0x3F, 0x41 - 0x46)"
      # "Start of Date Bytes"
      # "Store GIUD command:\n0x29:0x80:0x04:0x80:0x00:0x25:0x64:0x00:0x0B:0xXX:0xXX:0xXX:0xXX:0xXX:0xXX:0xXX:0xXX:0xXX:0xXX:0xXX:0xXX:0xXX:0xXX:0xXX:0xXX:0xXX:0xXX:0xXX:0xXX:0xXX:0xXX:0xXX:0xXX:0xXX:0xXX:0xXX:0xXX:0xXX:0xXX:0xXX:0xXX:"
      n171 = call "Generate GUID.vi"() -> ("GUID"=w506:string)  [unwired: 10 in, 1 out]
      "GUID" <- w506
      n172 = String To Byte Array(string=w506) -> (unsigned byte array=w503:u8[])
      n173 = Insert Into Array(array=u8[] [41, 128, 4, 128, 0, 37, 100, 0, 11], index=9, new element=w503) -> (w502:u8[])
    }
    frame "Cable Auto ID" {
      w509 = TRUE  # Get Response
      w510 = TRUE  # Get ACK/NAK
      # "0x05, 0xA1, 0x04, 0x00, 0x6E"
    }
    frame "Store RSM 627" {
      w512 = FALSE  # Get Response
      w513 = TRUE  # Get ACK/NAK
      # "0x0A, 0xA1, 0x04, 0x80, 0x45, 0x02, 0x73, 0x42, 0x07, 0x02"
    }
    frame "Hall Effect switch" {
      w515 = TRUE  # Get Response
      w516 = TRUE  # Get ACK/NAK
    }
    frame "Read RSM 627" {
      w519 = TRUE  # Get Response
      w518 = TRUE  # Get ACK/NAK
      # "\"0x07, 0xA1, 0x04, 0x80, 0x42,0x02,0x73\""
    }
  }
  n174 = case shown="False" FALSE {
    tunnel: [w521 w525] -> w8
    tunnel: [_ w524] -> w7
    tunnel: "VISA resource name" -> [w521 w522]
    frame False {
    }
    frame True {
      n175 = call "MIMIC Port Init.vi"("MIMIC TIMEOUT"=u32 500, "MIMC BAUD"=u32 9600, "MIMIC_PORT"=w522) -> ("error out"=w524:errorcluster, "MIMIC PORT RESOURCE"=w525:refnum<visa-resource-name>)
    }
  }
  n176 = local write "Array"(w6) -> ()
  n177 = call "XmitMIMICCommand.vi"("error in (no error)"=w7, "HWHSflag"="HWHSflag", "Command array"=w6, "VISA resource name"=w8) -> ("error out"=w22:errorcluster, "VISA resource name Out"=w21:refnum<visa-resource-name>)
  n178 = case shown="False" w27 {
    tunnel: [w529 w533] -> w26
    tunnel: w22 -> [w529 w538]
    tunnel: w21 -> [w528 w536]
    tunnel: [w528 w534] -> w24
    tunnel: [_ w532] -> w16
    tunnel: [w527 w531] -> w15
    tunnel: "wait (ms)" -> [w527 w530]
    frame False {
    }
    frame True {
      # "NEED TO CHECK ACK"
      n179 = flat-sequence {
        tunnel: w538 -> [w541]
        tunnel: [w541] -> w537
        tunnel: w536 -> [w540]
        tunnel: [w540] -> w535
        tunnel: [w539] -> w531
        tunnel: w530 -> [w539]
        tunnel: w537 -> [w546]
        tunnel: w535 -> [w545]
        tunnel: [w544] -> w534
        tunnel: [w543] -> w533
        tunnel: [w542] -> w532
        frame #0 {
          n180 = Wait (ms)(milliseconds to wait=w539) -> ()  [unwired: 1 out]
        }
        frame #1 {
          n181 = call "MIMIC RecvCommand.vi"("error in"=w546, "VISA resource name"=w545) -> ("error out"=w543:errorcluster, "Receive_buffer"=w542:u8[], "VISA resource name OUT"=w544:refnum<visa-resource-name>)  [unwired: 2 in, 1 out]
          n182 = Number To Hexadecimal String(2:w542) -> (0:→"hex integer string":string[])  [unwired: 1 in]
        }
      }
    }
  }
  n183 = case shown="True" w25 {
    tunnel: [w550 w557] -> w17
    tunnel: w26 -> [w550 w552]
    tunnel: w24 -> [w549 w554]
    tunnel: [w548 w558] -> w18
    tunnel: [w549 w556] -> w19
    tunnel: w16 -> [w548 _]
    tunnel: w15 -> [_ w551]
    frame False {
    }
    frame True {
      n184 = flat-sequence {
        tunnel: [w561] -> w555
        tunnel: w554 -> [w561]
        tunnel: [w560] -> w553
        tunnel: w552 -> [w560]
        tunnel: w551 -> [w559]
        tunnel: [w566] -> w558
        tunnel: [w565] -> w557
        tunnel: [w564] -> w556
        tunnel: w555 -> [w562]
        tunnel: w553 -> [w563]
        frame #0 {
          n185 = Wait (ms)(milliseconds to wait=w559) -> ()  [unwired: 1 out]
        }
        frame #1 {
          n186 = call "MIMIC RecvCommand.vi"("error in"=w563, "VISA resource name"=w562) -> ("error out"=w565:errorcluster, "Receive_buffer"=w566:u8[], "VISA resource name OUT"=w564:refnum<visa-resource-name>)  [unwired: 2 in, 1 out]
        }
      }
    }
  }
  n187 = case shown="\"General-Response\"" "MIMIC HOST COMMAND" {
    tunnel: w19 -> [w574 w578 w581 w584 w593 w596 w599 w602 w605 w608 w611 w614 w617 w620 w623 w626 w629 w632 w635 w647 w650 w653 w656 w659 w662 w671 w674 w681 w700 w723 w726 w732 w768 w804 w818 w832 w835 w837 w854 w859 w862 w866 w876 w887 w895 w898 w907 w909 w920 w931 w936 w954 w957 w960 w963 w968 w981]
    tunnel: [w574 w578 w581 w584 w593 w596 w599 w602 w605 w608 w611 w614 w617 w620 w623 w626 w629 w632 w635 w647 w650 w653 w656 w659 w662 w671 w674 w681 w700 w723 w726 w732 w768 w804 w818 w832 w835 w837 w854 w859 w862 w866 w876 w887 w895 w898 w907 w909 w920 w931 w936 w954 w957 w960 w963 w968 w981] -> w13
    tunnel: w18 -> [w570 w577 w580 w583 w585 w595 w598 w601 w604 w607 w610 w613 w616 w619 w622 w625 w628 w631 w634 w645 w649 w652 w655 w658 w661 w663 w673 w676 w698 w722 w725 w728 w737 w773 w809 w823 w833 w839 w849 w858 w863 w867 w873 w886 w892 w897 w904 w910 w916 w924 w933 w949 w956 w959 w962 w965 w980]
    tunnel: [w570 w577 w580 w583 w585 w595 w598 w601 w604 w607 w610 w613 w616 w619 w622 w625 w628 w631 w634 w640 w649 w652 w655 w658 w661 w663 w673 w675 w698 w722 w725 w727 w737 w773 w809 w823 w833 w838 w852 w858 w860 w867 w871 w886 w889 w897 w902 w910 w912 w922 w935 w948 w956 w959 w962 w964 w980] -> w12
    tunnel: w17 -> [w575 w576 w579 w582 w592 w594 w597 w600 w603 w606 w609 w612 w615 w618 w621 w624 w627 w630 w633 w646 w648 w651 w654 w657 w660 w670 w672 w680 w701 w721 w724 w731 w767 w803 w817 w831 w834 w836 w853 w857 w861 w868 w877 w885 w896 w899 w908 w911 w919 w932 w937 w953 w955 w958 w961 w967 w979]
    tunnel: [w575 w576 w579 w582 w592 w594 w597 w600 w603 w606 w609 w612 w615 w618 w621 w624 w627 w630 w633 w646 w648 w651 w654 w657 w660 w670 w672 w680 w701 w721 w724 w731 w767 w803 w817 w831 w834 w836 w853 w857 w861 w868 w877 w885 w896 w899 w908 w911 w919 w932 w937 w953 w955 w958 w961 w967 w979] -> w11
    tunnel: [w572 _ _ _ w586 _ _ _ _ _ _ _ _ _ _ _ _ _ _ w641 _ _ _ _ _ w667 _ _ w703 _ _ _ w738 w774 w805 w819 _ _ w850 _ _ _ w869 w879 w890 _ w900 _ w914 w923 _ w946 _ _ _ _ _] -> w9
    frame "Enter FAT", Default {
      n188 = Array Subset(array=w570, index=5, length=200) -> (w569:u8[])
      n189 = Byte Array To String(unsigned byte array=w569) -> (string=w573:string)
      n190 = local read "Receive_Unpacked_Data"() -> (w571:T1)
      n191 = Bundle By Name(cluster=w571, "Response_String_1"=w573) -> (w572:T1)
    }
    frame "Beeper Control" {
    }
    frame "ParamSend" {
    }
    frame "General" {
    }
    frame "General-Response" {
      n192 = Number To Hexadecimal String(1:i16 2 ("width (-)"), 2:w585) -> (0:w589:string[])
      n193 = local read "Receive_Unpacked_Data"() -> (w587:T1)
      n194 = Concatenate Strings(w589, "" ("string")) -> (w590:string)
      n195 = Bundle By Name(cluster=w587, "Response_String_1"=w590) -> (w586:T1)
    }
    frame "RSM Init" {
    }
    frame "RSM EnterFAT" {
    }
    frame "RSM - SE4500 - Peek PRISM Register GENERIC command" {
    }
    frame "RSM - SE4500 - Poke PRISM Register GENERIC command" {
    }
    frame "RSM - SE4500 - GENERIC command" {
    }
    frame "RSM - SE4500 - SetPDM Calibration" {
    }
    frame "RSM - SE4500 - SetPDM-Z Calibration" {
    }
    frame "LED On" {
    }
    frame "Image Mode" {
    }
    frame "Start Session" {
    }
    frame "Stop Session" {
    }
    frame "Change Buadrate" {
    }
    frame "Auto Exposure" {
    }
    frame "Set Manual Exposure" {
    }
    frame "Read BT Address" {
      n196 = Array Subset(array=w645, index=14, length=6) -> (w640:u8[])
      n197 = Number To Hexadecimal String(1:i16 2 ("width (-)"), 2:w640) -> (0:w638:string[])
      n198 = local read "Receive_Unpacked_Data"() -> (w642:T1)
      n199 = Concatenate Strings(w638, "" ("string")) -> (w637:string)
      n200 = Bundle By Name(cluster=w642, "Response_String_1"=w637) -> (w641:T1)
    }
    frame "Store BT Address" {
    }
    frame "Pairing Command" {
    }
    frame "Un-Pairing" {
    }
    frame "Set Illumination" {
    }
    frame "Set Defaults" {
    }
    frame "Exit FAT" {
      n201 = Array Subset(array=w663, index=5, length=13) -> (w664:u8[])
      n202 = Byte Array To String(unsigned byte array=w664) -> (string=w669:string)
      n203 = local read "Receive_Unpacked_Data"() -> (w668:T1)
      n204 = Bundle By Name(cluster=w668, "Response_String_1"=w669) -> (w667:T1)
    }
    frame "LED Off" {
    }
    frame "Trigger" {
      n205 = Empty Array?(array=w676) -> (empty?=w677:bool)
      n206 = case shown="False" w677 {
        tunnel: w676 -> [w683 _]
        tunnel: [w682 w689] -> w675
        frame False {
          n207 = Array Subset(array=w683, index=5, length=1) -> (w682:u8[])
        }
        frame True {
          # "If empty, init array and set its values to zero."
          n208 = To Unsigned Byte Integer(number=u8 0) -> (unsigned 8bit integer=w687:u8)
          n209 = Initialize Array(w687, 1 ("dimension size")) -> (w689:u8[])
        }
      }
      n210 = Array Subset(array=w676, index=5, length=1) -> ()  [unwired: 1 out]
    }
    frame "Imager Time To Decode Test" {
      n211 = Byte Array To String(unsigned byte array=w698) -> (string=w714:string)
      n212 = Replace Substring(2:16 ("length (len. of substring)"), 3:0 ("offset (0)"), 5:w714) -> (1:w709:string)  [unwired: 1 in, 1 out]
      n213 = String Length(string=w709) -> (length=w708:i32)
      n214 = Index Array(array=w698, index=5) -> (element=w711:u8)
      n215 = Subtract(x=w708, y=2) -> (x-y=w706:i32)
      n216 = Index Array(array=w698, index=7 ("length")) -> (element=w693:u8)
      n217 = Index Array(array=w698, index=6) -> (element=w696:u8)
      n218 = case shown="1" w711 {
        frame 0, Default {
          n219 = local read "Receive_Unpacked_Data"() -> (w715:T1)
          n220 = Bundle By Name(cluster=w715, "Decode_Status"="No Decode" ("Decode_Data")) -> (w716:T1)
          n221 = local write "Receive_Unpacked_Data"(w716) -> ()
        }
        frame 1 {
          n222 = local read "Receive_Unpacked_Data"() -> (w719:T1)
          n223 = Bundle By Name(cluster=w719, "Decode_Status"="SUCCESS" ("Decode_Data")) -> (w718:T1)
          n224 = local write "Receive_Unpacked_Data"(w718) -> ()
        }
      }
      n225 = Join Numbers(hi=u8 0, lo=w696) -> ((hi.lo)=w691:u16)
      n226 = Join Numbers(hi=w693, lo=u8 0 ("hi")) -> ((hi.lo)=w692:u16)
      n227 = Add(x=w691, y=w692) -> (x+y=w690:u16)
      n228 = local write "TimeToDecode"(w690) -> ()
      n229 = Replace Substring(2:2 ("length (len. of substring)"), 3:w706, 5:w709) -> (1:w704:string)  [unwired: 1 in, 1 out]
      n230 = local read "Receive_Unpacked_Data"() -> (w702:T1)
      n231 = Bundle By Name(cluster=w702, "Decode_Data"=w704, "Time_To_Decode"=w690) -> (w703:T1)
    }
    frame "Battery Off" {
    }
    frame "Battery Charge Control" {
    }
    frame "Read Battery Voltage" {
      # "Voltage (MSB_LSB *.0006*2)"
      # "RESPONSE\nLength Byte:\t0x0D\nOpcode Byte:\t0x21\nSource Byte:\t0x00\nStatus Byte:\t0x80\nSub-opcode Byte:\t0x42\nData Byte 1:\t0x75: Attribute MSB\nData Byte 2:\t0x30: Attribute LSB\nData Byte 3:\t0x57: Attribute is Word ('W') value\nData Byte 4:\t0x01\nData Byte 5:\t0xXX: Battery Voltage MSB\nData Byte 6:\t0xXX: Battery Voltage LSB\nData Byte 7:\t0xFF: Packet Termination\nData Byte 8:\t0xFF: Packet Termination\nChecksum High Byte:\t0xXX\nChecksum Low Byte:\t0xXX"
      n232 = Array Subset(array=w728, index=0, length=15) -> (w727:u8[])
    }
    frame "RSM - SE4500 - GetPDM Calibration" {
      n233 = Index Array(array=w737, index=14) -> (element=w763:u8)
      n234 = Index Array(array=w737, index=16) -> (element=w756:u8)
      n235 = Index Array(array=w737, index=13) -> (element=w764:u8)
      n236 = Index Array(array=w737, index=15) -> (element=w757:u8)
      n237 = Index Array(array=w737, index=18) -> (element=w749:u8)
      n238 = Index Array(array=w737, index=20) -> (element=w743:u8)
      n239 = Index Array(array=w737, index=17) -> (element=w750:u8)
      n240 = Index Array(array=w737, index=19) -> (element=w744:u8)
      n241 = Join Numbers(hi=w763, lo=w764) -> ((hi.lo)=w736:u16)
      n242 = Join Numbers(hi=w756, lo=w757) -> ((hi.lo)=w733:u16)
      n243 = Join Numbers(hi=w749, lo=w750) -> ((hi.lo)=w734:u16)
      n244 = Join Numbers(hi=w743, lo=w744) -> ((hi.lo)=w735:u16)
      n245 = Number To Decimal String(number=w736, width (-)=i16 4) -> (decimal integer string=w762:string)
      n246 = Number To Decimal String(number=w733, width (-)=i16 4) -> (decimal integer string=w755:string)
      n247 = Number To Decimal String(number=w734, width (-)=i16 4) -> (decimal integer string=w748:string)
      n248 = Number To Decimal String(number=w735, width (-)=i16 4) -> (decimal integer string=w742:string)
      n249 = local read "Receive_Unpacked_Data"() -> (w760:T1)
      n250 = Bundle By Name(cluster=w760, "Response_String_1"=w762) -> (w753:T1)
      n251 = Bundle By Name(cluster=w753, "Response_String_2"=w755) -> (w740:T1)
      n252 = Bundle By Name(cluster=w740, "Response_String_3"=w748) -> (w739:T1)
      n253 = Bundle By Name(cluster=w739, "Response_String_4"=w742) -> (w738:T1)
    }
    frame "RSM - SE4500 - GetPDM-Z Calibration" {
      n254 = Index Array(array=w773, index=14) -> (element=w799:u8)
      n255 = Index Array(array=w773, index=16) -> (element=w792:u8)
      n256 = Index Array(array=w773, index=13) -> (element=w800:u8)
      n257 = Index Array(array=w773, index=15) -> (element=w793:u8)
      n258 = Index Array(array=w773, index=22) -> (element=w785:u8)
      n259 = Index Array(array=w773, index=24) -> (element=w779:u8)
      n260 = Index Array(array=w773, index=21) -> (element=w786:u8)
      n261 = Index Array(array=w773, index=23) -> (element=w780:u8)
      n262 = Join Numbers(hi=w799, lo=w800) -> ((hi.lo)=w772:u16)
      n263 = Join Numbers(hi=w792, lo=w793) -> ((hi.lo)=w769:u16)
      n264 = Join Numbers(hi=w785, lo=w786) -> ((hi.lo)=w770:u16)
      n265 = Join Numbers(hi=w779, lo=w780) -> ((hi.lo)=w771:u16)
      n266 = Number To Decimal String(number=w772, width (-)=i16 4) -> (decimal integer string=w798:string)
      n267 = Number To Decimal String(number=w769, width (-)=i16 4) -> (decimal integer string=w791:string)
      n268 = Number To Decimal String(number=w770, width (-)=i16 4) -> (decimal integer string=w784:string)
      n269 = Number To Decimal String(number=w771, width (-)=i16 4) -> (decimal integer string=w778:string)
      n270 = local read "Receive_Unpacked_Data"() -> (w796:T1)
      n271 = Bundle By Name(cluster=w796, "Response_String_1"=w798) -> (w789:T1)
      n272 = Bundle By Name(cluster=w789, "Response_String_2"=w791) -> (w776:T1)
      n273 = Bundle By Name(cluster=w776, "Response_String_3"=w784) -> (w775:T1)
      n274 = Bundle By Name(cluster=w775, "Response_String_4"=w778) -> (w774:T1)
    }
    frame "Get Object Sensor Value" {
      n275 = Index Array(array=w809, index=5) -> (element=w808:u8)
      n276 = Index Array(array=w809, index=6) -> (element=w807:u8)
      n277 = Number To Hexadecimal String(1:i16 2 ("width (-)"), 2:w808) -> (0:w816:string)
      n278 = Number To Hexadecimal String(1:i16 2 ("width (-)"), 2:w807) -> (0:w812:string)
      n279 = local read "Receive_Unpacked_Data"() -> (w814:T1)
      n280 = Bundle By Name(cluster=w814, "Response_String_1"=w816) -> (w810:T1)
      n281 = Bundle By Name(cluster=w810, "Response_String_2"=w812) -> (w805:T1)
    }
    frame "Read Object Sensor Calibration Value" {
      n282 = Index Array(array=w823, index=9) -> (element=w822:u8)
      n283 = Index Array(array=w823, index=10) -> (element=w821:u8)
      n284 = Number To Hexadecimal String(1:i16 2 ("width (-)"), 2:w822) -> (0:w830:string)
      n285 = Number To Hexadecimal String(1:i16 2 ("width (-)"), 2:w821) -> (0:w826:string)
      n286 = local read "Receive_Unpacked_Data"() -> (w828:T1)
      n287 = Bundle By Name(cluster=w828, "Response_String_1"=w830) -> (w824:T1)
      n288 = Bundle By Name(cluster=w824, "Response_String_2"=w826) -> (w819:T1)
    }
    frame "Store Object Sensor Calibration Value" {
    }
    frame "Read Battery Temperature" {
      # "RESPONSE\nLength Byte:\t0x0D\nOpcode Byte:\t0x21\nSource Byte:\t0x00\nStatus Byte:\t0x80\nSub-opcode Byte:\t0x42\nData Byte 1:\t0x75: Attribute MSB\nData Byte 2:\t0x31: Attribute LSB\nData Byte 3:\t0x57: Attribute is Word ('W') value\nData Byte 4:\t0x01\nData Byte 5:\t0xXX: Battery Temperature MSB\nData Byte 6:\t0xXX: Battery Temperature LSB\nData Byte 7:\t0xFF: Packet Termination\nData Byte 8:\t0xFF: Packet Termination\nChecksum High Byte:\t0xXX\nChecksum Low Byte:\t0xXX"
      n289 = Array Subset(array=w839, index=0, length=15) -> (w838:u8[])
    }
    frame "Software Version" {
      n290 = Array Subset(array=w849, index=32, length=16) -> (w846:u8[])
      n291 = Array Subset(array=w849, index=13, length=16) -> (w852:u8[])
      n292 = Byte Array To String(unsigned byte array=w852) -> (string=w845:string)
      n293 = Byte Array To String(unsigned byte array=w846) -> (string=w844:string)
      n294 = Concatenate Strings(w845, "  " ("string"), w844) -> (w842:string)
      n295 = local read "Receive_Unpacked_Data"() -> (w851:T1)
      n296 = Bundle By Name(cluster=w851, "Code_Revision"=w842) -> (w850:T1)
    }
    frame "StoreFeatureSet" {
    }
    frame "ReadFeatureSet" {
      # "Feature Set Responce:\n0x0C, 0x21, 0x00, 0x00, 0x42, 0x02, 0xC2,0x42,0x01,\n\t\t\t\t\t\t\t\t\t\t\t  \t\t\t  0xff, //FEATURE-SET\n\t\t\t\t\t\t\t\t\t\t\t\t\t\t  0xff,0xff, // packet termination\n\t\t\t\t\t\t\t\t\t\t\t\t\t\t  0x00, 0x00}; //checksum"
      n297 = Array Subset(array=w863, index=9, length=1) -> (w860:u8[])
    }
    frame "Store Model Number" {
    }
    frame "Read Model Number" {
      n298 = Array Subset(array=w873, index=13, length=18) -> (w871:u8[])
      n299 = Byte Array To String(unsigned byte array=w871) -> (string=w872:string)
      n300 = local read "Receive_Unpacked_Data"() -> (w870:T1)
      n301 = Bundle By Name(cluster=w870, "Response_String_1"=w872) -> (w869:T1)
    }
    frame "Store Manufacturing Date" {
      n302 = Get Date/Time In Seconds() -> (seconds since 1Jan1904=w884:timestamp)
      n303 = Format Date/Time String(time format string (%c)="%d%b%y", seconds (now)=w884, UTC format=FALSE) -> (date/time string=w881:string)
      n304 = To Upper Case(1:w881) -> (0:w878:string)
      n305 = local read "Receive_Unpacked_Data"() -> (w880:T1)
      n306 = Bundle By Name(cluster=w880, "Response_String_1"=w878) -> (w879:T1)
    }
    frame "Read Manufacturing Date" {
      n307 = Array Subset(array=w892, index=13, length=7) -> (w889:u8[])
      n308 = Byte Array To String(unsigned byte array=w889) -> (string=w891:string)
      n309 = local read "Receive_Unpacked_Data"() -> (w888:T1)
      n310 = Bundle By Name(cluster=w888, "Response_String_1"=w891) -> (w890:T1)
    }
    frame "Store Service Date" {
    }
    frame "Read Service Date" {
      n311 = Array Subset(array=w904, index=13, length=7) -> (w902:u8[])
      n312 = Byte Array To String(unsigned byte array=w902) -> (string=w903:string)
      n313 = local read "Receive_Unpacked_Data"() -> (w901:T1)
      n314 = Bundle By Name(cluster=w901, "Response_String_1"=w903) -> (w900:T1)
    }
    frame "Store Serial Number" {
    }
    frame "Read Serial Number" {
      n315 = Array Subset(array=w916, index=13, length=16) -> (w912:u8[])
      n316 = Byte Array To String(unsigned byte array=w912) -> (string=w915:string)
      n317 = local read "Receive_Unpacked_Data"() -> (w913:T1)
      n318 = Bundle By Name(cluster=w913, "Response_String_1"=w915) -> (w914:T1)
    }
    frame "Query Paired Address" {
      # "Cradle BT Address"
      # "Pair Status\n0x00: Unpaired \n0x01: Paired"
      n319 = Array Subset(array=w924, index=6, length=6) -> (w927:u8[])
      n320 = Array Subset(array=w924, index=5, length=1) -> (w922:u8[])
      n321 = local read "Receive_Unpacked_Data"() -> (w921:T1)
      n322 = Byte Array To String(unsigned byte array=w927) -> (string=w928:string)
      n323 = Bundle By Name(cluster=w921, "Response_String_1"=w928) -> (w923:T1)
    }
    frame "Pairing Status" {
      # "Pairing Status\n0x00: Cradle is not paired\n0x01: Cradle is paired"
      n324 = Empty Array?(array=w933) -> (empty?=w934:bool)
      n325 = case shown="False" w934 {
        tunnel: w933 -> [w939 _]
        tunnel: [w938 w945] -> w935
        frame False {
          n326 = Array Subset(array=w939, index=5, length=1) -> (w938:u8[])
        }
        frame True {
          # "If empty, init array and set its values to zero."
          n327 = To Unsigned Byte Integer(number=u8 0) -> (unsigned 8bit integer=w943:u8)
          n328 = Initialize Array(w943, 1 ("dimension size")) -> (w945:u8[])
        }
      }
    }
    frame "Read GUID" {
      n329 = Array Subset(array=w949, index=5, length=32) -> (w948:u8[])
      n330 = Byte Array To String(unsigned byte array=w948) -> (string=w952:string)
      n331 = local read "Receive_Unpacked_Data"() -> (w947:T1)
      n332 = Bundle By Name(cluster=w947, "Response_String_1"=w952) -> (w946:T1)
    }
    frame "Cable Auto ID" {
    }
    frame "Store RSM 627" {
    }
    frame "Store GUID " {
    }
    frame "Hall Effect switch" {
      n333 = Empty Array?(array=w965) -> (empty?=w966:bool)
      n334 = case shown="True" w966 {
        tunnel: w965 -> [w972 _]
        tunnel: [w971 w978] -> w964
        frame False {
          n335 = Array Subset(array=w972, index=5, length=1) -> (w971:u8[])
        }
        frame True {
          # "If empty, init array and set its values to zero."
          n336 = To Unsigned Byte Integer(number=u8 0) -> (unsigned 8bit integer=w976:u8)
          n337 = Initialize Array(w976, 1 ("dimension size")) -> (w978:u8[])
        }
      }
      n338 = Array Subset(array=w965, index=5, length=1) -> ()  [unwired: 1 out]
    }
    frame "Read RSM 627" {
    }
  }
  "error out" <- w11
  "Receive_buffer" <- w12
  "VISA resource name OUT" <- w13
  "Receive_Unpacked_Data" <- w9
  "TimeToDecode" <- u16 0 ("TimeToDecode")
